vi "Bank.vi"() -> ()   [LabVIEW 2013]
doc: "Ce VI simule les transactions effectuées dans une banque. Il est utilisé par un exercice du cours LabVIEW Fondamental 1 pour démontrer les conditions de compétition.\n\nExécutez le VI et faites deux transactions simultanément ; vous remarquerez que l'une des transactions (débit ou crédit) est perdue. Essayez de trouver la source du problème et de corriger l'erreur."
panel:
  out "Solde":dbl
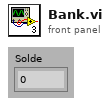
[diagram p1: front panel]
types:
  T1 = typedef "Account Info.ctl" = cluster{"Rendez-vous Banque":T2, "File d'attente des débits":refnum<queue>, "File d'attente des crédits":refnum<queue>}
  T2 = typedef "Rendezvous RefNum" = refnum<k1>
  T3 = typedef "Semaphore RefNum" = refnum<k1>
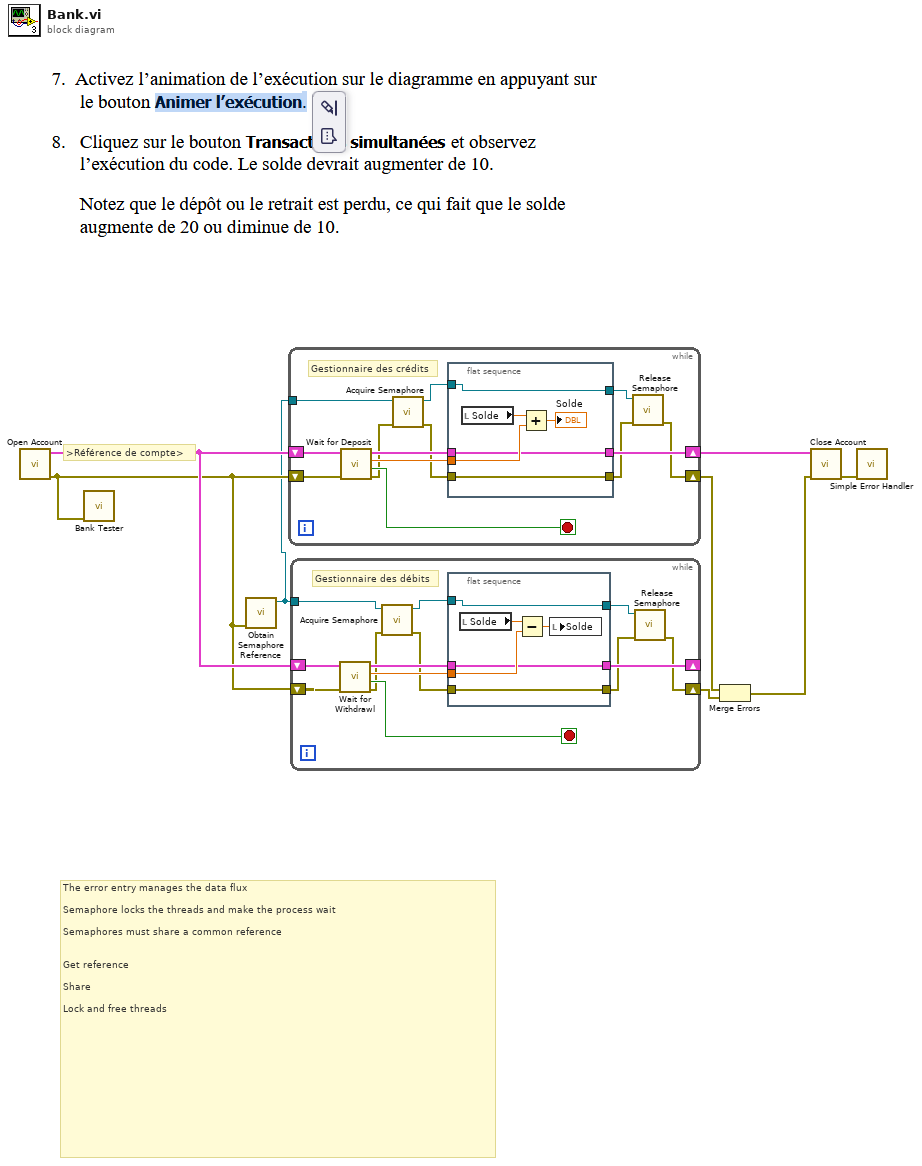
[diagram p0: block diagram]
diagram:
  # "The error entry manages the data flux\n\nSemaphore locks the threads and make the process wait\n\nSemaphores must share a common reference\n\n\nGet reference\n\nShare\n\nLock and free threads"
  # ">Référence de compte>"
  n1 = call "Open Account.vi"() -> ("sortie d'erreur"=w2:errorcluster, "Infos sur le compte"=w8:T1)  [unwired: 10 out]
  n2 = call "Bank Tester.vi"("entrée d'erreur (pas d'erreur)"=w2) -> ()  [unwired: 11 out]
  n3 = call <vilib>:"Obtain Semaphore Reference.vi"("error in (no error)"=w2) -> ("semaphore"=w1:T3)  [unwired: 4 in, 2 out]
  n4 = while "Boucle While" {
    shift-right: [w17] -> w5
    shift-left: w8 -> [w20]
    shift-right: [w12] -> w7
    shift-left: w2 -> [w19]
    tunnel: w1 -> [w11]
    stop <- w16 stop-if-true
    # "Gestionnaire des crédits"
    n5 = call "Wait for Deposit.vi"("entrée d'erreur (pas d'erreur)"=w19, "Infos sur le compte"=w20) -> ("sortie d'erreur"=w15:errorcluster, "Arrêter ?"=w16:bool, "Montant à créditer"=w21:dbl, "Infos sur le compte en sortie"=w18:T1)  [unwired: 6 out]
    n6 = call <vilib>:"Acquire Semaphore.vi"("error in (no error)"=w15, "semaphore"=w11) -> ("error out"=w14:errorcluster, "semaphore out"=w10:T3)  [unwired: 3 in, 1 out]
    n7 = flat-sequence {
      tunnel: w21 -> [w27]
      tunnel: [w24] -> w17
      tunnel: w18 -> [w24]
      tunnel: w14 -> [w23]
      tunnel: [w23] -> w13
      tunnel: w10 -> [w22]
      tunnel: [w22] -> w9
      frame #0 {
        n8 = local read "Solde"() -> (w25:dbl)
        n9 = Add(x=w25, y=w27) -> (x+y=→"Solde":dbl)
      }
    }
    n10 = call <vilib>:"Release Semaphore.vi"("error in (no error)"=w13, "semaphore"=w9) -> ("error out"=w12:errorcluster)  [unwired: 4 in, 1 out]
  }
  n11 = while "Boucle While" {
    shift-right: [w36] -> _
    shift-left: w8 -> [w39]
    shift-right: [w31] -> w6
    shift-left: w2 -> [w38]
    tunnel: w1 -> [w30]
    stop <- w35 stop-if-true
    # "Gestionnaire des débits"
    n12 = call "Wait for Withdrawl.vi"("entrée d'erreur (pas d'erreur)"=w38, "Infos sur le compte"=w39) -> ("sortie d'erreur"=w34:errorcluster, "Arrêter ?"=w35:bool, "Montant à débiter"=w40:dbl, "Infos sur le compte en sortie"=w37:T1)  [unwired: 6 out]
    n13 = call <vilib>:"Acquire Semaphore.vi"("error in (no error)"=w34, "semaphore"=w30) -> ("error out"=w33:errorcluster, "semaphore out"=w29:T3)  [unwired: 3 in, 1 out]
    n14 = flat-sequence {
      tunnel: w40 -> [w44]
      tunnel: w37 -> [w43]
      tunnel: w33 -> [w42]
      tunnel: [w43] -> w36
      tunnel: [w42] -> w32
      tunnel: w29 -> [w41]
      tunnel: [w41] -> w28
      frame #0 {
        n15 = local read "Solde"() -> (w45:dbl)
        n16 = Subtract(x=w45, y=w44) -> (x-y=w46:dbl)
        n17 = local write "Solde"(w46) -> ()
      }
    }
    n18 = call <vilib>:"Release Semaphore.vi"("error in (no error)"=w32, "semaphore"=w28) -> ("error out"=w31:errorcluster)  [unwired: 4 in, 1 out]
  }
  n19 = Merge Errors(w7, w6) -> (w3:errorcluster)
  n20 = call "Close Account.vi"("entrée d'erreur"=w3, "Infos sur le compte"=w5) -> ("sortie d'erreur"=w4:errorcluster)  [unwired: 9 out]
  n21 = call <vilib>:"Simple Error Handler.vi"("error in (no error)"=w4) -> ()  [unwired: 1 in, 8 out]
